vi "GetMatlabCOM.vi"(1 "MatlabCOM":string, 2 "Mode":enum16{"Initialize", "Run"}(ring)) -> (0 "ParsedCOM":T1)   [LabVIEW 2011]
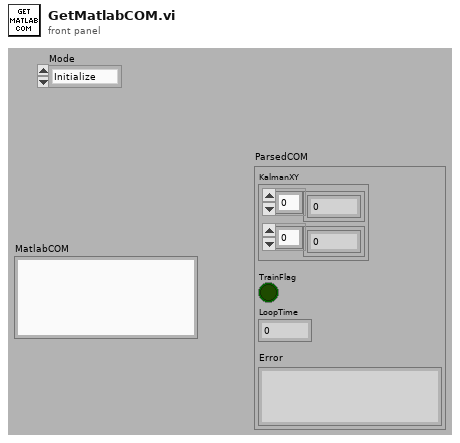
[diagram p1: front panel]
types:
  T1 = cluster{"Error":string, "KalmanXY":cluster{dbl[], dbl[]}, "TrainFlag":bool, "LoopTime":dbl}
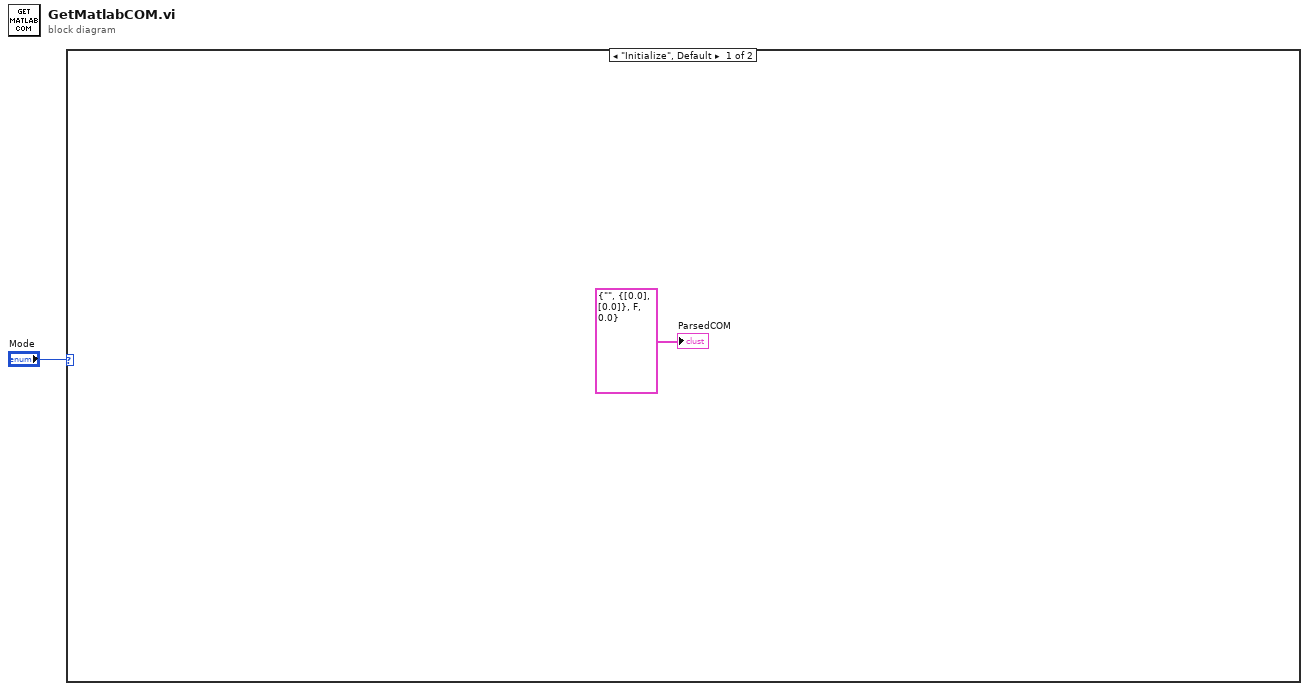
[diagram p0: block diagram]
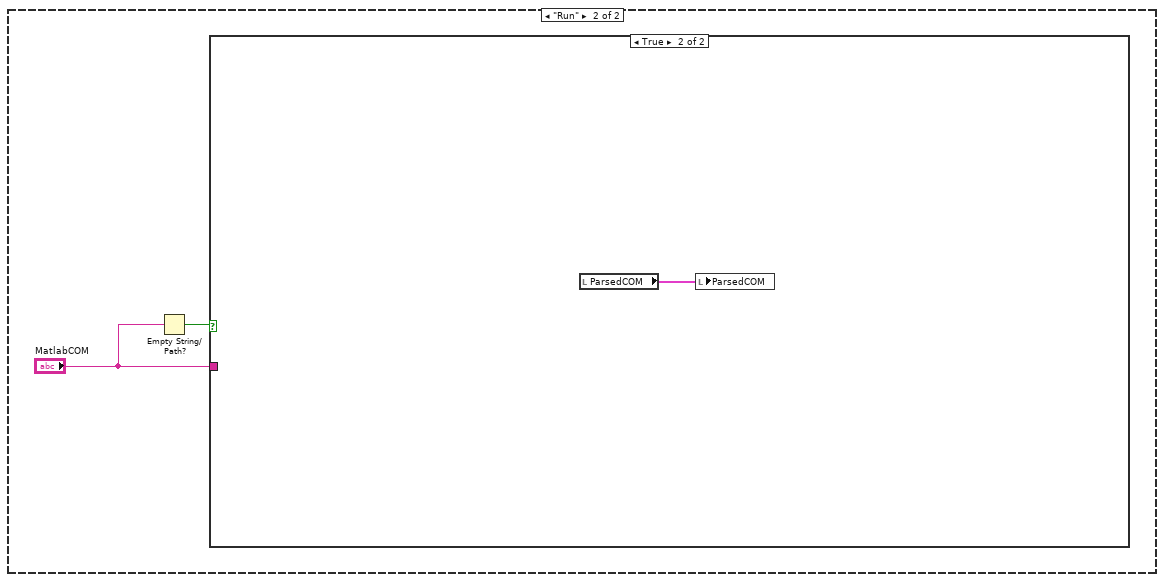
[diagram p2: hidden frame]
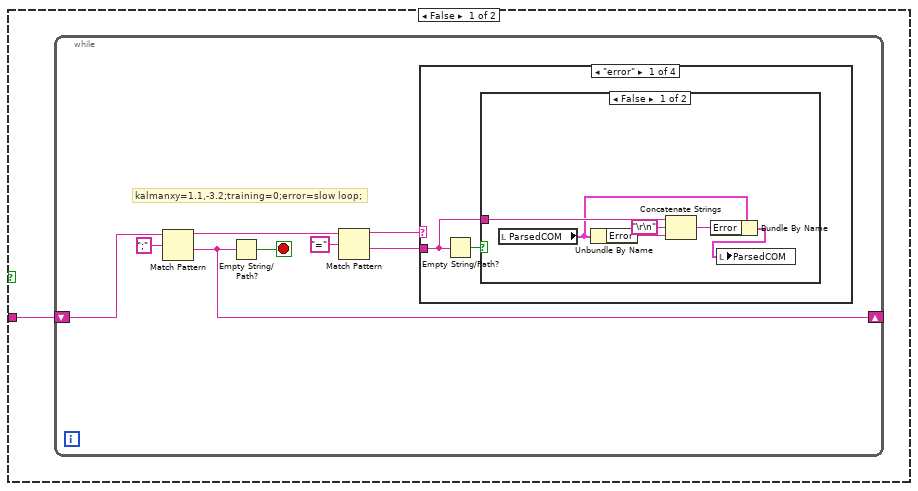
[diagram p3: hidden frame]
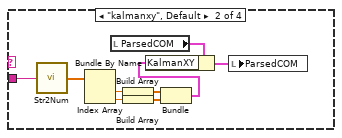
[diagram p5: hidden frame]
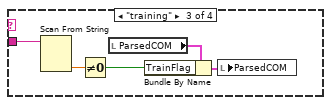
[diagram p6: hidden frame]
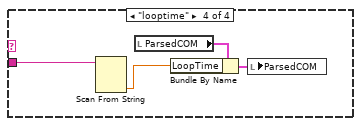
[diagram p7: hidden frame]
diagram:
  n1 = case shown="\"Initialize\", Default" "Mode" {
    frame "Initialize", Default {
      "ParsedCOM" <- T1 {"Error"="", "KalmanXY"={[0.0], [0.0]}, "TrainFlag"=FALSE, "LoopTime"=0.0} ("ParsedCOM")
    }
    frame "Run" {
      n2 = Empty String/Path?(string/path="MatlabCOM") -> (empty?=w3:bool)
      n3 = case shown="True" w3 {
        tunnel: "MatlabCOM" -> [w5 _]
        frame False {
          n4 = while {
            shift-right: [w10] -> _
            shift-left: w5 -> [w11]
            stop <- w12 stop-if-true
            # "kalmanxy=1.1,-3.2;training=0;error=slow loop;"
            n5 = Match Pattern(string=w11, regular expression=";") -> (before substring=w9:string, after substring=w10:string)  [unwired: 1 in, 2 out]
            n6 = Empty String/Path?(string/path=w10) -> (empty?=w12:bool)
            n7 = Match Pattern(string=w9, regular expression="=") -> (before substring=w7:string, after substring=w6:string)  [unwired: 1 in, 2 out]
            n8 = case shown="\"error\"" w7 {
              tunnel: w6 -> [w14 w30 w34 w39]
              frame "error" {
                n9 = Empty String/Path?(string/path=w14) -> (empty?=w15:bool)
                n10 = case shown="False" w15 {
                  tunnel: w14 -> [w20 _]
                  frame False {
                    n11 = local read "ParsedCOM"() -> (w19:T1)
                    n12 = Unbundle By Name(w19) -> ("Error"=w17:string)
                    n13 = Concatenate Strings(w20, "\r\n", w17) -> (w16:string)
                    n14 = Bundle By Name(cluster=w19, "Error"=w16) -> (w21:T1)
                    n15 = local write "ParsedCOM"(w21) -> ()
                  }
                  frame True {
                  }
                }
              }
              frame "kalmanxy", Default {
                n16 = call "Str2Num.vi"("InputString"=w30) -> ("Array"=w23:dbl[])
                n17 = Index Array(array=w23) -> (element #1=w27:dbl, element #2=w26:dbl)  [unwired: 2 in]
                n18 = local read "ParsedCOM"() -> (w29:T1)
                n19 = Build Array(w27) -> (w25:dbl[])
                n20 = Build Array(w26) -> (w24:dbl[])
                n21 = Bundle(w25, w24) -> (w22:cluster{dbl[], dbl[]})  [unwired: 1 in]
                n22 = Bundle By Name(cluster=w29, "KalmanXY"=w22) -> (w28:T1)
                n23 = local write "ParsedCOM"(w28) -> ()
              }
              frame "training" {
                n24 = Scan From String(input string=w34) -> (output 1=w32:dbl)  [unwired: 4 in, 3 out]
                n25 = Not Equal To 0?(x=w32) -> (x != 0?=w31:bool)
                n26 = local read "ParsedCOM"() -> (w35:T1)
                n27 = Bundle By Name(cluster=w35, "TrainFlag"=w31) -> (w33:T1)
                n28 = local write "ParsedCOM"(w33) -> ()
              }
              frame "looptime" {
                n29 = Scan From String(input string=w39) -> (output 1=w36:dbl)  [unwired: 4 in, 3 out]
                n30 = local read "ParsedCOM"() -> (w38:T1)
                n31 = Bundle By Name(cluster=w38, "LoopTime"=w36) -> (w37:T1)
                n32 = local write "ParsedCOM"(w37) -> ()
              }
            }
          }
        }
        frame True {
          n33 = local read "ParsedCOM"() -> (w40:T1)
          n34 = local write "ParsedCOM"(w40) -> ()
        }
      }
    }
  }
